vi "to string.vi"(8 "error in":errorcluster, 11 "fixed channel configuration in":refnum<class "ScaleAndLimitModule configuration.lvclass">) -> (0 "error out":errorcluster, 1 "data":string, 2 "version":string, 3 "fixed channel configuration out":refnum<class "ScaleAndLimitModule configuration.lvclass">)   [LabVIEW 2017, in "ScaleAndLimitModule configuration.lvclass"]
doc: "Provides an interface for saving a module configuration to a file or other serialized data source. It is recommended that all children of this class store data in two sets--data required for its own initialization, and any data required for parent initialization--and that each implementation uses the <b>Call Parent Method</b> primitive to serialize parent information.\nNI Tag Bus Module Framework 1.0.3.43\nNI Systems Engineering"
uses:
  ScaleAndLimitModule configuration.lvclass
  ScaleAndLimitModule configuration.lvclass/ScaleAndLimitModule configuration.ctl
  <vilib>/NI/DCAF/Tag Editor Core/control module/configuration/control module configuration.lvclass
  <vilib>/NI/Configuration Framework/serializable configuration/NISE_CEF_serializable configuration.lvclass
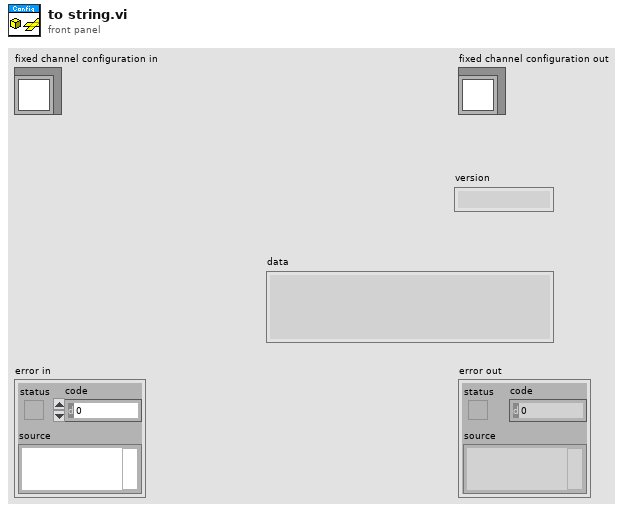
[diagram p1: front panel]
types:
  T1 = typedef "ScaleAndLimitInterface.lvlib/Configuration.ctl" = cluster{"Name":string, "M":dbl, "B":i16, "HighLimit":dbl, "LowLimit":dbl, "LimitsEnabled":bool}
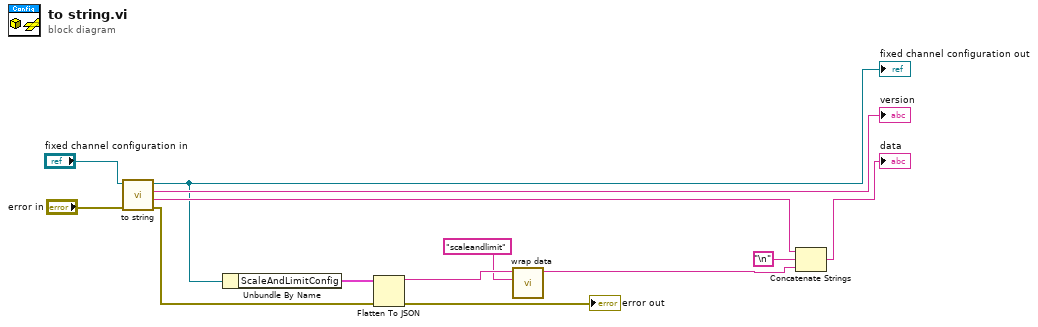
[diagram p0: block diagram]
diagram:
  n1 = call-parent "to string.vi"("error in"="error in", "fixed channel configuration in"="fixed channel configuration in") -> ("error out"=w2:errorcluster, "data"=w10:string, "version"=→"version":string, "fixed channel configuration out"=w7:refnum<class "ScaleAndLimitModule configuration.lvclass">)  [unwired: 6 in]
  "fixed channel configuration out" <- w7
  n2 = Unbundle By Name(w7) -> ("ScaleAndLimitConfig"=w6:T1[])
  n3 = Flatten To JSON(anything=w6, error in (no error)=w2) -> (JSON string=w5:string, 11:→"error out":errorcluster)  [unwired: 1 in]
  n4 = call <vilib>:"wrap data.vi"("identifier"="scaleandlimit", "data to wrap"=w5) -> ("wrapped data"=w3:string)  [unwired: 9 in]
  n5 = Concatenate Strings(w10, "\n", w3) -> (→"data":string)
